vi "save_image.vi"(9 "Image index":u32) -> ()   [LabVIEW 2011]
uses:
  Action-Init-Update-Get.ctl
  <userlib>/atmcd32d.llb/Tiff_type typedef.ctl
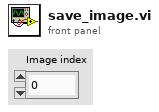
[diagram p1: front panel]
types:
  T1 = typedef "Action-Init-Update-Get.ctl" = enum16{"Initialize", "Update", "Get"}
  T2 = typedef "Tiff_type typedef.ctl" = enum16{"8-bit", "16-bit", "color"}
  T3 = cluster{"Path":string, "Filestem":string, "Filestem incl time t":string, "Date":string}
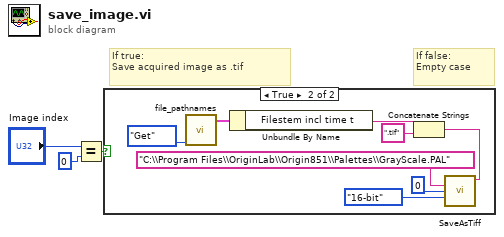
[diagram p0: block diagram]
diagram:
  # "If false:\nEmpty case"
  # "If true:\nSave acquired image as .tif"
  n1 = Equal?(x="Image index", y=u32 0) -> (x = y?=w1:bool)
  n2 = case shown="True" w1 {
    frame False {
    }
    frame True {
      n3 = call "file_pathnames.vi"("Action"=Action-Init-Update-Get."Get") -> ("File-path\n-names"=w8:T3)  [unwired: 10 in]
      n4 = Unbundle By Name(w8) -> ("Filestem incl time t"=w6:string)
      n5 = Concatenate Strings(w6, ".tif" ("string")) -> (w5:string)
      n6 = call <userlib>:"SaveAsTiff.vi"("path"=w5, "palette"="C:\\Program Files\\OriginLab\\Origin851\\Palettes\\GrayScale.PAL", "position"=0, "type"=Tiff_type_typedef."16-bit") -> ()  [unwired: 10 in, 2 out]
    }
  }
